vi "MSEditor_SaveScriptFile_new.vi"(2 "script":string, 3 "path_str":string) -> (0 "error out":errorcluster, 1 "dup_path_str":string)   [LabVIEW 2018]
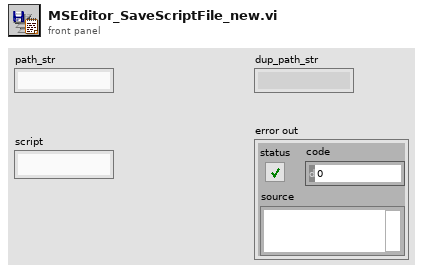
[diagram p1: front panel]
types:
  T1 = enum16{"open", "replace", "create", "open or create", "replace or create", "replace or create with confirmation"}
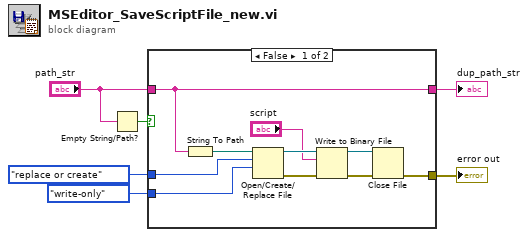
[diagram p0: block diagram]
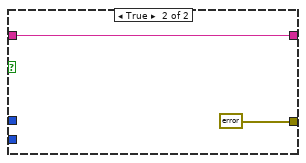
[diagram p2: hidden frame]
diagram:
  n1 = Empty String/Path?(string/path="path_str") -> (empty?=w6:bool)
  n2 = case shown="False" w6 {
    tunnel: "path_str" -> [w7 w17]
    tunnel: [w7 w17] -> w4
    tunnel: T1."replace or create" ("operation (0:open)") -> [w13 _]
    tunnel: enum16{"read/write", "read-only", "write-only"}."write-only" ("access (0:read/write)") -> [w12 _]
    tunnel: [w8 errorcluster {"status"=TRUE, "code"=5200, "source"="Write Failed , Please confirm the path is  correct."} ("error out")] -> w1
    frame False {
      n3 = String To Path(string=w7) -> (path=w14:path)
      n4 = Open/Create/Replace File(file path (use dialog)=w14, operation (0:open)=w13, access (0:read/write)=w12) -> (refnum out=w11:refnum<file>, error out=w15:errorcluster)  [unwired: 3 in, 1 out]
      n5 = Write to Binary File(file (use dialog)=w11, data="script", error in=w15) -> (refnum out=w10:refnum<file>, error out=w16:errorcluster)  [unwired: 3 in, 1 out]
      n6 = Close File(refnum=w10, error in=w16) -> (error out=w8:errorcluster)  [unwired: 1 out]
    }
    frame True {
    }
  }
  "dup_path_str" <- w4
  "error out" <- w1
